vi "102_LabOneNodes.vi"() -> ()   [LabVIEW 2009]
uses:
  <instrlib>/Zurich Instruments LabOne/Public/Configure/ziGetValueString.vi
  <instrlib>/Zurich Instruments LabOne/Zurich Instruments LabOne.lvlib
panel:
  out "Tab Control":T1(tab)
  in  "Flags":T2
  out "Nodes":string[](array[string])
  out "# of Nodes HF2":i32
  out "Doc":T3(array[cluster])
  in  "Flags":T4
  out "# of Nodes":i32
  in  "Path (\"\")":string
  in  "stop":bool
  out "Connected?":bool
  in  "Address":string="DEV"
  out "Error Out":errorcluster
  # "LabOne Nodes\nAll communication with an instrument occurs via the Data Server program the instrument is connected to. The Data Server organizes the instrument's settings and data in a file-system-like hierarchical structure called the node tree. This VI provides the list of these nodes. Except for the HF2 Instruments, you can also see the node descriptions.   \n\nYou can find more on the nodes, their properties and types in the LabOne programming manual: \nhttps://docs.zhinst.com//labone_programming_manual/instrument_communication.html#commons.nodedoc.tree\n\nRequirements: Any Zurich Instrument Product\n\n\nTo run:\n1- Type the Instrument ID \n2- Run the VI\n3- Update the path \n\nTested Devices:\n- HF2LI\n- UHFLI\n- MFLI\n\n\n\n\n(c) Zurich Instruments.  ALL RIGHTS RESERVED."
  # "HF2 Instruments\nThe data server that handles communication with HF2 Instruments (ziServer. exe) provides the nodes' list. The LabVIEW API can call this list with the ziList.vi utility function. \n\nIt lists the highest node hierarchy if the Path control is empty. You can look into the inner nodes by entering a note path listed. For the node properties and types, you can refer to the user manual: \n\nhttps://docs.zhinst.com/labone_programming_manual/instrument_communication.html#commons.nodedoc.exploringnodes\n\nNote: ziServer.exe does not provide node documentation, which is available for other Zurich Instruments products."
  # "LabOne Data server\nThe Data Server that handles communication with the instrument, ziDataServer.exe, provides the node documentation using the ziListNodesJSON.vi utility function. \n\nYou can see the node's description, properties, type, and unit. For enumerated nodes, you can also see the options possible to set.\n \nFor the node properties and types, you can refer to the user manual: \nhttps://docs.zhinst.com/labone_programming_manual/instrument_communication.html#commons.nodedoc.exploringnodes"
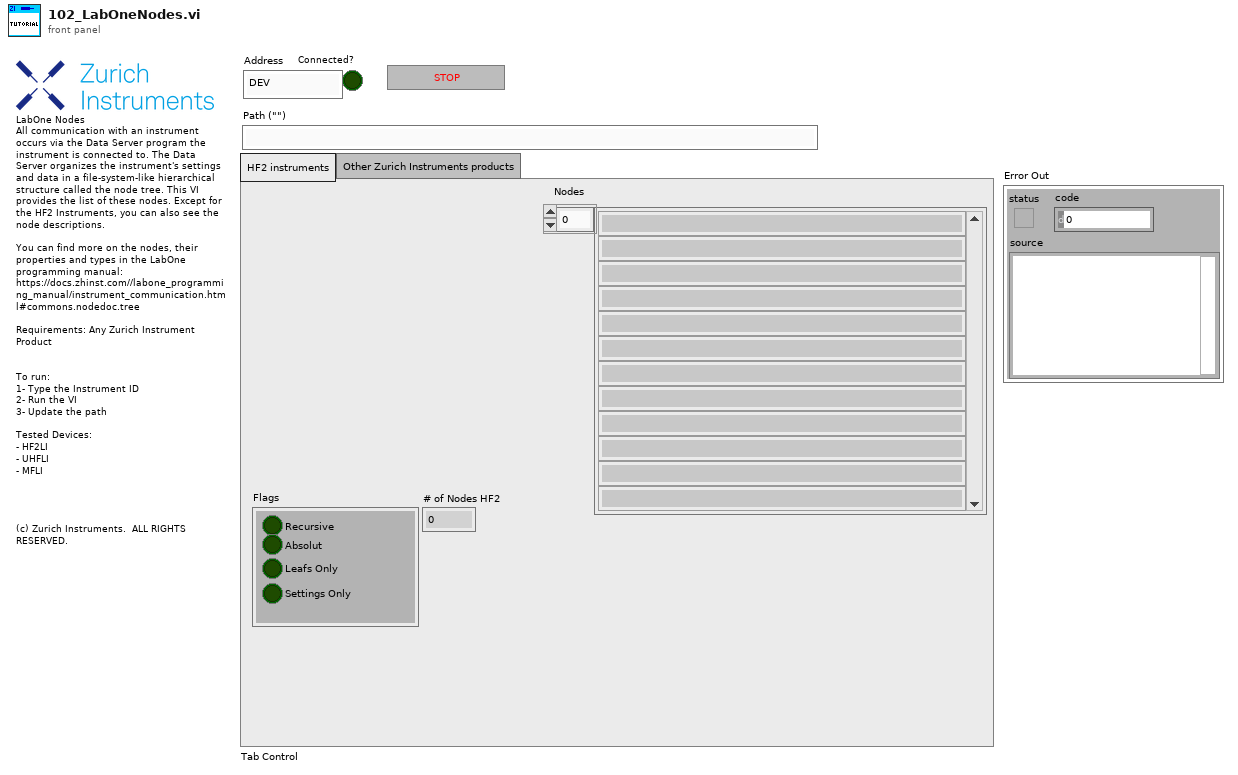
[diagram p1: front panel]
types:
  T1 = enum32{"HF2 instruments", "Other Zurich Instruments products"}
  T2 = cluster{"Recursive":bool, "Absolut":bool, "Leafs Only":bool, "Settings Only":bool}
  T3 = cluster{"Node":string, "Description":string, "Properties":string, "Type":string, "Unit":string, "Options":string}[]
  T4 = cluster{"Recursive":bool, "Absolut":bool, "Leafs Only":bool, "Settings Only":bool, "Streaming Only":bool, "Subscribe Only":bool}
  T5 = typedef "Zurich Instruments LabOne.lvlib/ziTypeHandle.ctl" = cluster{"handleValid":bool, "Conn":u64, "Path Prefix":string, "Handle":u64, "Connected":bool, "Clockbase(s)":dbl}
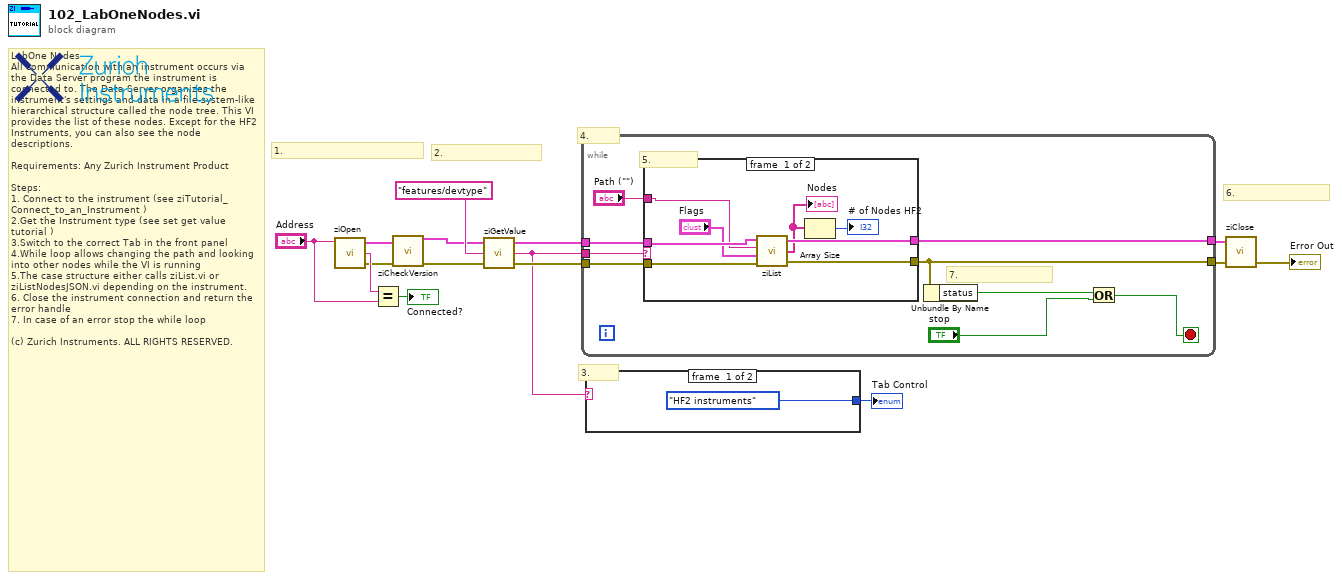
[diagram p0: block diagram]
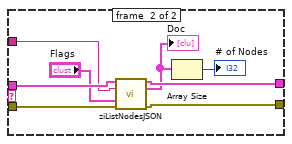
[diagram p2: hidden frame]
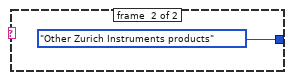
[diagram p3: hidden frame]
diagram:
  # "6."
  # "4."
  # "3."
  # "2."
  # "1."
  # "LabOne Nodes\nAll communication with an instrument occurs via the Data Server program the instrument is connected to. The Data Server organizes the instrument's settings and data in a file-system-like hierarchical structure called the node tree. This VI provides the list of these nodes. Except for the HF2 Instruments, you can also see the node descriptions. \n\nRequirements: Any Zurich Instrument Product\n\nSteps:\n1. Connect to the instrument (see ziTutorial_Connect_to_an_Instrument )\n2.Get the Instrument type (see set get value tutorial )\n3.Switch to the correct Tab in the front panel\n4.While loop allows changing the path and looking into other nodes while the VI is running\n5.The case structure either calls ziList.vi or ziListNodesJSON.vi depending on the instrument.   \n6. Close the instrument connection and return the error handle \n7. In case of an error stop the while loop \n\n(c) Zurich Instruments. ALL RIGHTS RESERVED."
  n1 = call <instrlib>:"ziOpen.vi"("Address"="Address") -> ("Error Out"=w12:errorcluster, "Selected Device"=w14:string, "HandleOut"=w13:T5)  [unwired: 1 in, 2 out]
  n2 = Equal?(x=w14, y="Address") -> (x = y?=→"Connected?":bool)
  n3 = call <instrlib>:"ziCheckVersion.vi"("Handle In"=w13, "Error In"=w12) -> ("Handle Out"=w8:T5, "Error Out"=w7:errorcluster)  [unwired: 11 in, 1 out]
  n4 = call-poly <instrlib>:"ziGetValue.vi"("error in"=w7, "Path"="features/devtype", "Handle In"=w8) -> ("error out"=w5:errorcluster, "Value"=w2:string, "Handle Out"=w6:T5)
  n5 = while {
    tunnel: w2 -> [w24]
    tunnel: w6 -> [w22]
    tunnel: w5 -> [w21]
    tunnel: [w19] -> w4
    tunnel: [w20] -> w3
    stop <- w17 stop-if-true
    # "7."
    # "5."
    n6 = case shown="Default" w24 {
      tunnel: "Path (\"\")" -> [w28 w35]
      tunnel: w22 -> [w32 w40]
      tunnel: w21 -> [w31 w37]
      tunnel: [w30 w38] -> w19
      tunnel: [w29 w39] -> w20
      frame #0 {
        n7 = call <instrlib>:"ziList.vi"("Error In"=w31, "Flags (None)"="Flags", "Path (\"\")"=w28, "Handle In"=w32) -> ("Error Out"=w30:errorcluster, "Nodes"=w26:string[], "Handle Out"=w29:T5)
        "Nodes" <- w26
        n8 = Array Size(array=w26) -> (size(s)=→"# of Nodes HF2":i32)
      }
      frame #1 {
        n9 = call <instrlib>:"ziListNodesJSON.vi"("Handle In"=w40, "Path (\"\")"=w35, "Flags (None)"="Flags", "Error In"=w37) -> ("Handle Out"=w39:T5, "Doc"=w34:T3, "Error Out"=w38:errorcluster)  [unwired: 9 in]
        "Doc" <- w34
        n10 = Array Size(array=w34) -> (size(s)=→"# of Nodes":i32)
      }
    }
    n11 = Unbundle By Name(w19) -> ("status"=w18:bool)
    n12 = Or(x=w18, y="stop") -> (x .or. y?=w17:bool)
  }
  n13 = case shown="\"HF2IS\", \"HF2LI\"" w2 {
    tunnel: [T1."HF2 instruments" ("Tab Control") T1."Other Zurich Instruments products" ("Tab Control")] -> w1
    frame #0 {
    }
    frame #1 {
    }
  }
  "Tab Control" <- w1
  n14 = call <instrlib>:"ziClose.vi"("Error In"=w4, "Handle In"=w3) -> ("Error Out"=→"Error Out":errorcluster)  [unwired: 2 in, 1 out]
